vi "worker_VAR.vi"(4 "IN VARIANT":variant) -> (1 "OUT VARIANT":variant, 2 "Boolean":bool)   [LabVIEW 2015]
panel:
  in  "Iterations":i32=6000
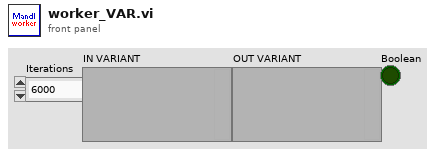
[diagram p1: front panel]
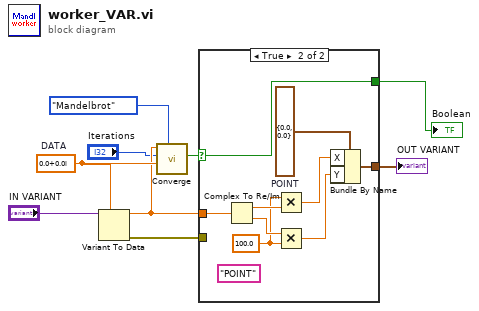
[diagram p0: block diagram]
diagram:
  w9 = cdb 0.0+0.0i  # DATA
  n1 = Variant To Data(type=w9, Variant="IN VARIANT") -> (data=w8:cdb, error out=w7:errorcluster)  [unwired: 1 in]
  n2 = call "Converge.vi"("Fractal type"=enum16{"Mandelbrot", "Julia"}."Mandelbrot", "Z0"=w9, "Iterations"="Iterations", "C"=w8) -> ("IN"=w6:bool)  [unwired: 6 in, 1 out]
  n3 = case shown="True" w6 {
    selector: w6 -> [_ w10]
    tunnel: w8 -> [_ w18]
    tunnel: w7 -> [_ _]
    tunnel: [_ w11] -> w2
    tunnel: [_ w10] -> w1
    frame False {
    }
    frame True {
      (unwired) "POINT" ("Name in")
      w12 = cluster{"X":dbl, "Y":dbl} {"X"=0.0, "Y"=0.0}  # POINT
      w15 = 100.0 ("x")
      n4 = Complex To Re/Im(x + iy=w18) -> (x=w17:dbl, y=w16:dbl)
      n5 = Multiply(x=w15, y=w17) -> (x*y=w14:dbl)
      n6 = Multiply(x=w16, y=w15) -> (x*y=w13:dbl)
      n7 = Bundle By Name(cluster=w12, "X"=w14, "Y"=w13) -> (w11:cluster{"X":dbl, "Y":dbl})
    }
  }
  "OUT VARIANT" <- w2
  "Boolean" <- w1
